vi "Get Column Data from Spreadsheet.vi"(10 "Column Tag":string="<TestName>", 11 "SpreadSheet Data In":string[][](array[string])) -> (3 "Column Data":string[](array[string]))   [LabVIEW 2018, in "Test Number and Bin Generator.lvlib" / "Test Number and Bin Generator.lvclass"]
uses:
  Test Number and Bin Generator.lvclass
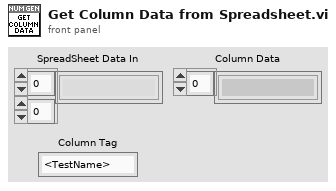
[diagram p1: front panel]
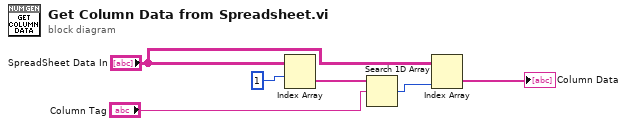
[diagram p0: block diagram]
diagram:
  n1 = Index Array(array="SpreadSheet Data In", index (row)=1) -> (element=w4:string[])  [unwired: 1 in]
  n2 = Search 1D Array(1D array=w4, element="Column Tag") -> (index of element=w2:i32)  [unwired: 1 in]
  n3 = Index Array(array="SpreadSheet Data In", index (col)=w2) -> (element=→"Column Data":string[])  [unwired: 1 in]
